vi "Untitled 2.vi"() -> ()   [LabVIEW 2015]
uses:
  Analog Output Channel/Analog Output Channel/Analog Output Channel.lvclass
  <vilib>/ActorFramework/Actor/Actor.lvclass
  Channel Messages/Open FP Msg/Open FP Msg.lvclass
panel:
  out "error out":errorcluster
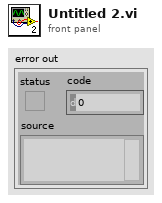
[diagram p1: front panel]
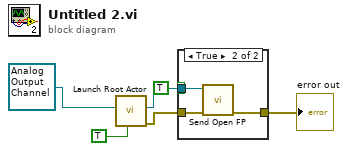
[diagram p0: block diagram]
diagram:
  n1 = call <vilib>:"Launch Root Actor.vi"("Open Actor Core front panel? (F)"=TRUE, "Actor"=refnum<class "Analog Output Channel.lvclass"> refnum ("Analog Output Channel.lvlib:Analog Output Channel.lvclass")) -> ("error out"=w4:errorcluster, "Actor's Enqueuer"=w5:refnum<class "Message Enqueuer.lvclass">)  [unwired: 8 in]
  n2 = case shown="True" TRUE {
    tunnel: w5 -> [_ w10]
    tunnel: w4 -> [w7 w9]
    tunnel: [w7 w8] -> w3
    frame False {
    }
    frame True {
      n3 = call "Send Open FP.vi"("error in (no error)"=w9, "Message Enqueuer in"=w10) -> ("error out"=w8:errorcluster)  [unwired: 8 in, 1 out]
    }
  }
  "error out" <- w3
